vi "Get File Info.vi"(11 "EDS in":refnum<class "EDS.lvclass">) -> (2 "File Info":refnum<class "File Info.lvclass">, 3 "EDS out":refnum<class "EDS.lvclass">)   [LabVIEW 2024, in "EDS.lvlib" / "EDS.lvclass"]
uses:
  EDS.lvclass
  EDS.lvclass/EDS.ctl
  File Info/File Info.lvclass
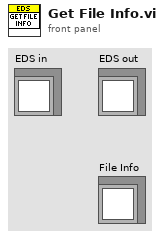
[diagram p1: front panel]
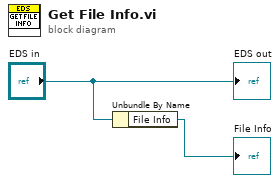
[diagram p0: block diagram]
diagram:
  n1 = Unbundle By Name("EDS in") -> ("File Info"=→"File Info":refnum<class "File Info.lvclass">)
  "EDS out" <- "EDS in"
